vi "display.get.vi"(11 "Worder in":refnum<class "Worder.lvclass">) -> (1 "keyboard":T1={"A"={"color"=3815996, "char"="A"}, "B"={"color"=3815996, "char"="B"}, "C"={"color"=3815996, "char"="C"}, "D"={"color"=3815996, "char"="D"}, "E"={"color"=3815996, "char"="E"}, "F"={"color"=3815996, "char"="F"}, "G"={"color"=3815996, "char"="G"}, "H"={"color"=3815996, "char"="H"}, "I"={"color"=3815996, "char"="I"}, "J"={"color"=3815996, "char"="J"}, "K"={"color"=3815996, "char"="K"}, "L"={"color"=3815996, "char"="L"}, "M"={"color"=3815996, "char"="M"}, "N"={"color"=3815996, "char"="N"}, "O"={"color"=3815996, "char"="O"}, "P"={"color"=3815996, "char"="P"}, "Q"={"color"=3815996, "char"="Q"}, "R"={"color"=3815996, "char"="R"}, "S"={"color"=3815996, "char"="S"}, "T"={"color"=3815996, "char"="T"}, "U"={"color"=3815996, "char"="U"}, "V"={"color"=3815996, "char"="V"}, "W"={"color"=3815996, "char"="W"}, "X"={"color"=3815996, "char"="X"}, "Y"={"color"=3815996, "char"="Y"}, "Z"={"color"=3815996, "char"="Z"}}, 2 "gameboard":T3[][](array[typedef]), 3 "Worder out":refnum<class "Worder.lvclass">)   [LabVIEW 2020, in "Worder.lvclass"]
uses:
  Worder.lvclass
  letter_box.ctl
  keyboard.ctl
  letter_box_small.ctl
  Worder.lvclass/Worder.ctl
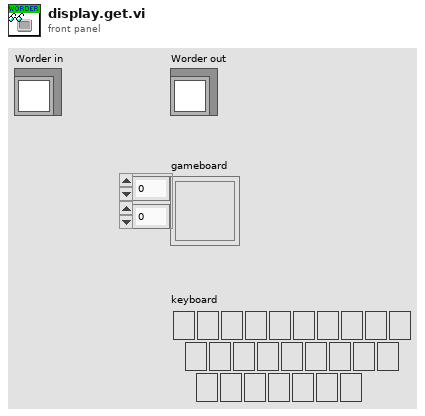
[diagram p1: front panel]
types:
  T1 = typedef "Worder.lvclass/keyboard.ctl" = cluster{"A":T2, "B":T2, "C":T2, "D":T2, "E":T2, "F":T2, "G":T2, "H":T2, "I":T2, "J":T2, "K":T2, "L":T2, "M":T2, "N":T2, "O":T2, "P":T2, "Q":T2, "R":T2, "S":T2, "T":T2, "U":T2, "V":T2, "W":T2, "X":T2, "Y":T2, "Z":T2}
  T2 = typedef "Worder.lvclass/letter_box_small.ctl" = cluster{"color":u32, "char":string}
  T3 = typedef "Worder.lvclass/letter_box.ctl" = cluster{"color":u32, "char":string}
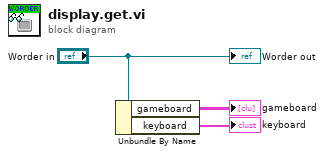
[diagram p0: block diagram]
diagram:
  n1 = Unbundle By Name("Worder in") -> ("gameboard"=→"gameboard":T3[][], "keyboard"=→"keyboard":T1)
  "Worder out" <- "Worder in"
